vi "TimeSpin.vi"(1 "x":i32, 2 "布尔":bool) -> (0 "activite":u16(ring))   [LabVIEW 2019]
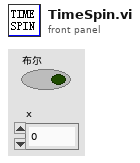
[diagram p1: front panel]
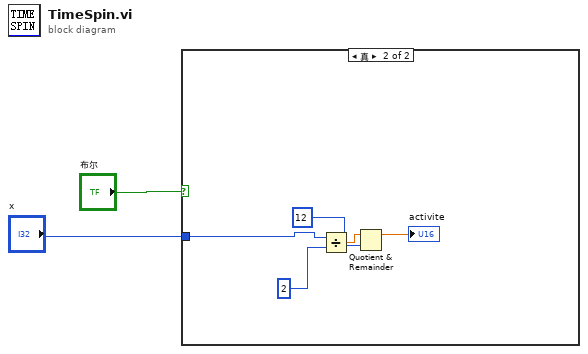
[diagram p0: block diagram]
diagram:
  n1 = case shown="真" "布尔" {
    tunnel: "x" -> [_ w3]
    frame False {
    }
    frame True {
      n2 = Divide(x=w3, y=2) -> (x/y=w4:dbl)
      n3 = Quotient & Remainder(x=w4, y=12) -> (x-y*floor(x/y)=→"activite":dbl)  [unwired: 1 out]
    }
  }
